vi "array_mean_double.vi"(1 "Input":dbl[](array[numeric])) -> (0 "Array Mean":dbl)   [LabVIEW 2019]
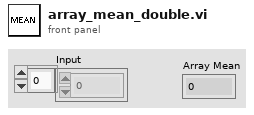
[diagram p1: front panel]
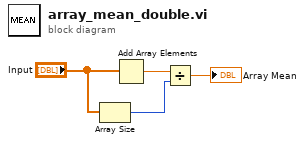
[diagram p0: block diagram]
diagram:
  n1 = Array Size(array="Input") -> (size(s)=w2:i32)
  n2 = Add Array Elements(numeric array="Input") -> (sum=w4:dbl)
  n3 = Divide(x=w4, y=w2) -> (x/y=→"Array Mean":dbl)
